vi "PanTompkinsAlg.vi"(1 "samplingFreq":dbl format="%0.2f", 2 "Signal":dbl[](array[numeric])) -> (0 "processedSignal":waveform(dbl))   [LabVIEW 2023]
uses:
  <vilib>/Analysis/3filter.llb/Filter Passband Type.ctl
  <vilib>/Analysis/3filter.llb/Butterworth Filter (DBL).vi
  <vilib>/addons/Time Series Analysis/Series Preprocess.llb/TSA Moving Average (Waveform).vi
  <vilib>/Analysis/NI_AALBase.lvlib
  <vilib>/addons/_Advanced Signal Processing/NI_AdvSigProcTSA.lvlib
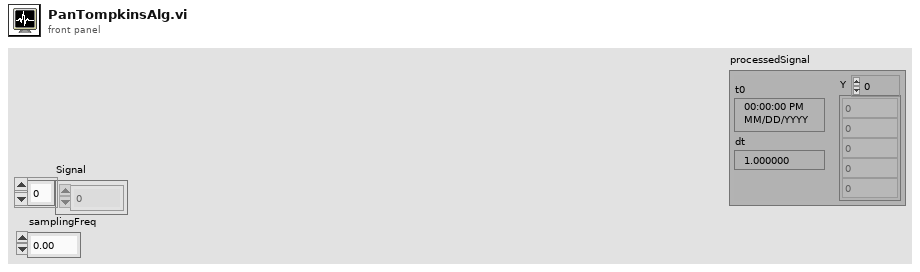
[diagram p1: front panel]
types:
  T1 = typedef "NI_AALBase.lvlib/Filter Passband Type.ctl" = enum32{"Lowpass", "Highpass", "Bandpass", "Bandstop"}
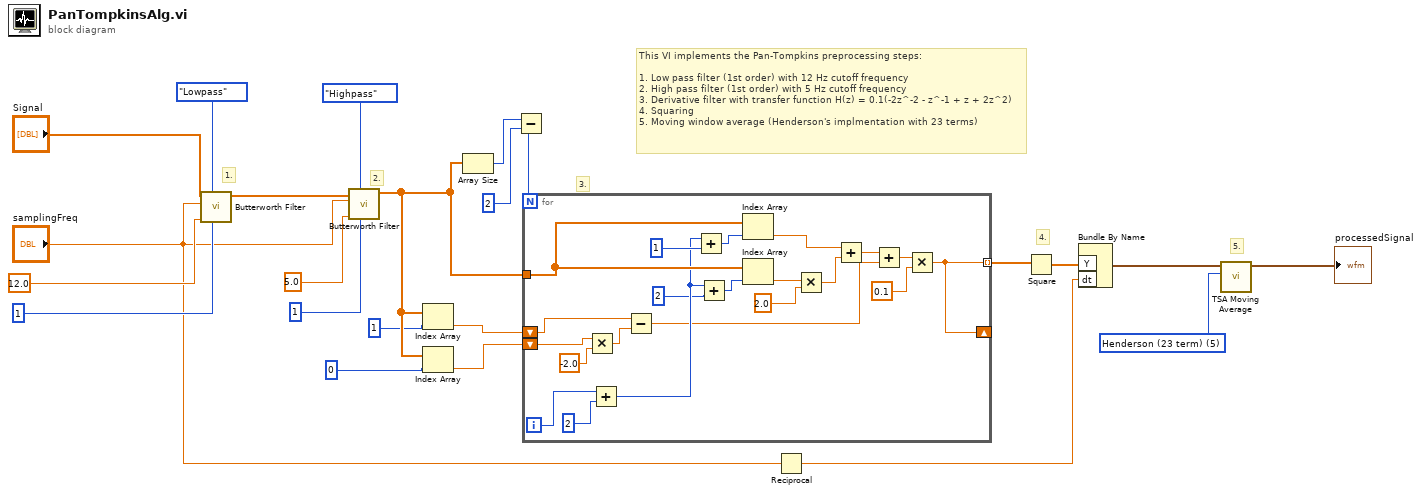
[diagram p0: block diagram]
diagram:
  w6 = 5 items=["Spencer (15 term)"=1, "Henderson (7 term)"=2, "Henderson (9 term)"=3, "Henderson (13 term)"=4, "Henderson (23 term)"=5] ("method")
  # "This VI implements the Pan-Tompkins preprocessing steps:\n\n1. Low pass filter (1st order) with 12 Hz cutoff frequency\n2. High pass filter (1st order) with 5 Hz cutoff frequency\n3. Derivative filter with transfer function H(z) = 0.1(-2z^-2 - z^-1 + z + 2z^2)\n4. Squaring\n5. Moving window average (Henderson's implmentation with 23 terms)"
  # "5."
  # "4."
  # "3."
  # "2."
  # "1."
  n1 = call-poly <vilib>:"Butterworth Filter.vi"("order"=1, "filter type"=Filter_Passband_Type."Lowpass", "low cutoff freq: fl"=12.0, "sampling freq: fs"="samplingFreq", "X"="Signal") -> ("Filtered X"=w19:dbl[])  [unwired: 3 in, 1 out]
  n2 = call-poly <vilib>:"Butterworth Filter.vi"("order"=1, "filter type"=Filter_Passband_Type."Highpass", "low cutoff freq: fl"=5.0, "sampling freq: fs"="samplingFreq", "X"=w19) -> ("Filtered X"=w15:dbl[])  [unwired: 3 in, 1 out]
  n3 = Index Array(array=w15, index=1) -> (element=w12:dbl)
  n4 = Index Array(array=w15, index=0) -> (element=w11:dbl)
  n5 = Array Size(array=w15) -> (size(s)=w10:i32)
  n6 = Subtract(x=w10, y=2) -> (x-y=w8:i32)
  n7 = for {
    N: w8 -> [_]
    tunnel: w15 -> [w38]
    shift-right: [w24] -> _
    shift-left: w12 -> [w39]
    shift-left: w11 -> [w41]
    tunnel: [w24] -> w7 mode=indexing
    i -> [w44]
    n8 = Multiply(x=w41, y=-2.0) -> (x*y=w40:dbl)
    n9 = Add(x=w44, y=2) -> (x+y=w34:i32)
    n10 = Subtract(x=w39, y=w40) -> (x-y=w27:dbl)
    n11 = Add(x=w34, y=i64 1) -> (x+y=w37:i64)
    n12 = Add(x=w34, y=2) -> (x+y=w35:i32)
    n13 = Index Array(array=w38, index=w37) -> (element=w29:dbl)
    n14 = Index Array(array=w38, index=w35) -> (element=w32:dbl)
    n15 = Multiply(x=w32, y=2.0) -> (x*y=w30:dbl)
    n16 = Add(x=w29, y=w30) -> (x+y=w28:dbl)
    n17 = Add(x=w28, y=w27) -> (x+y=w26:dbl)
    n18 = Multiply(x=w26, y=0.1) -> (x*y=w24:dbl)
  }
  n19 = Reciprocal(x="samplingFreq") -> (1/x=w3:dbl)
  n20 = Square(x=w7) -> (x^2=w5:dbl[])
  n21 = Bundle By Name("Y"=w5, "dt"=w3) -> (w2:waveform(dbl))  [unwired: 1 in]
  n22 = call-poly <vilib>:"TSA Moving Average.vi"("method"=w6, "Xt"=w2) -> ("Xt out"=→"processedSignal":waveform(dbl))  [unwired: 8 in, 1 out]
